vi "SwerveAntiDrift.vi"(1 "Max Driver Translation Joystick":dbl, 3 "Driver Rotation Joystick":dbl, 6 "PID Tuning Parameters":T1={"Kp"=0.1, "Ki"=0.1, "Kd"=0.1, "N-Diff"=10, "N-Int"=20, "Int Error Window"=0.5, "Max Ouput"=1.0, "Min Output"=-1.0, "Square Derivative"=FALSE, "N-Prop"=1} {"N-Prop" min=1; "Int Error Window" min=0.0; "N-Int" min=2; "N-Diff" min=2; "Kd" min=0.0; "Ki" min=0.0; "Kp" min=0.0}, 8 "Deceleration Hysteresis (ms)":u32, 10 "Strafe Deadband (ft/s)":dbl, 12 "External Disables":bool) -> (14 "Controller Summary":T2(graph), 17 "Joystick Rotation":dbl, 19 "Anti-Drift":bool)   [LabVIEW 2020]
doc: "This VI runs a PID controller to maintain the robot's heading while translating above a specified velocity. Dropping below the velocity threshold or manually commanding a rotation will switch off the anti-drift heading lock. Assumes that all of the joystick deadbands and scalings have already been applied."
uses:
  Globals/Sensor_Values.vi
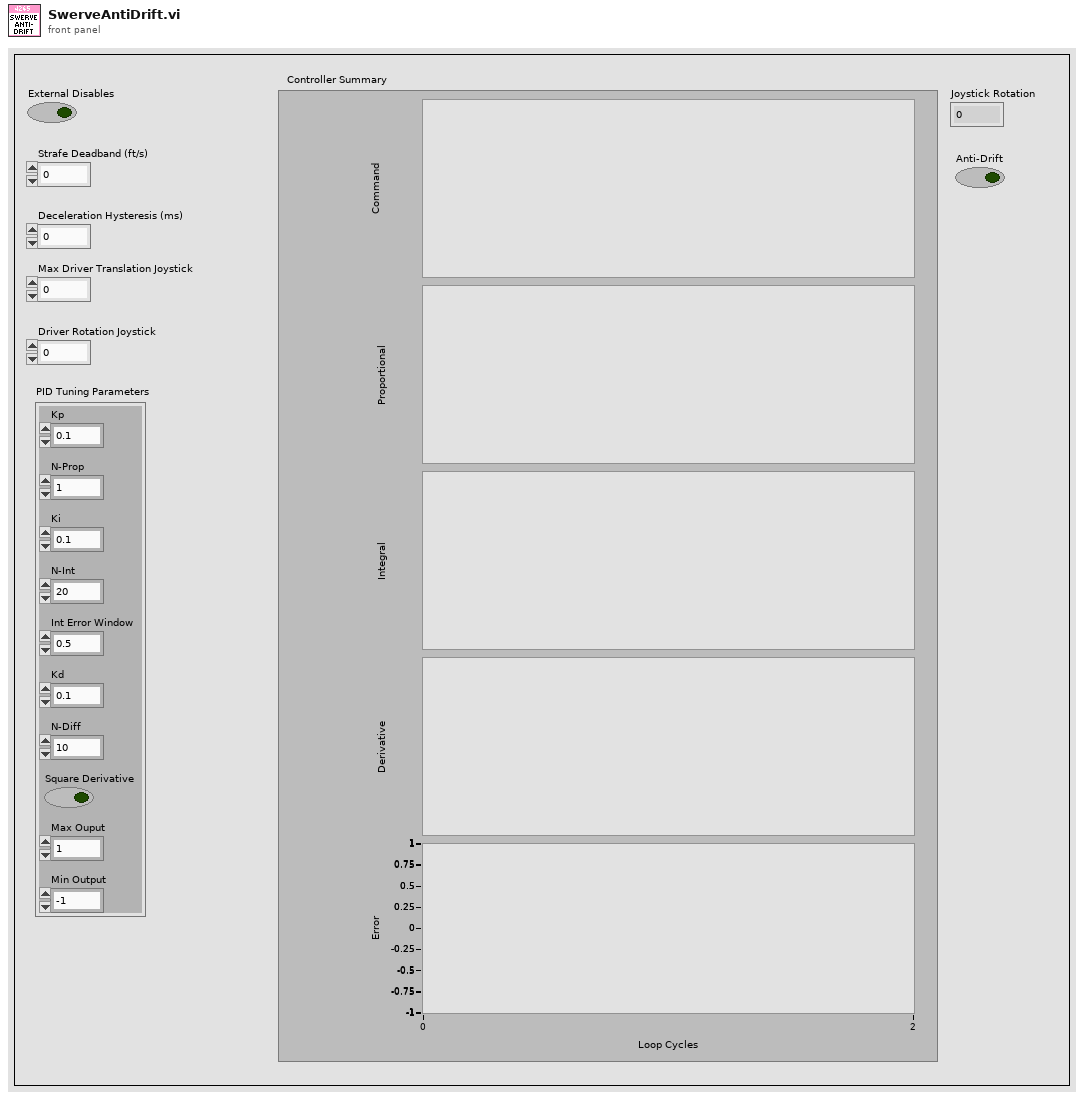
[diagram p1: front panel]
types:
  T1 = cluster{"Kp":dbl, "Ki":dbl, "Kd":dbl, "N-Diff":i32, "N-Int":i32, "Int Error Window":dbl, "Max Ouput":dbl, "Min Output":dbl, "Square Derivative":bool, "N-Prop":i32}
  T2 = cluster{"Command":dbl, "Proportional":dbl, "Integral":dbl, "Derivative":dbl, "Goal":dbl}
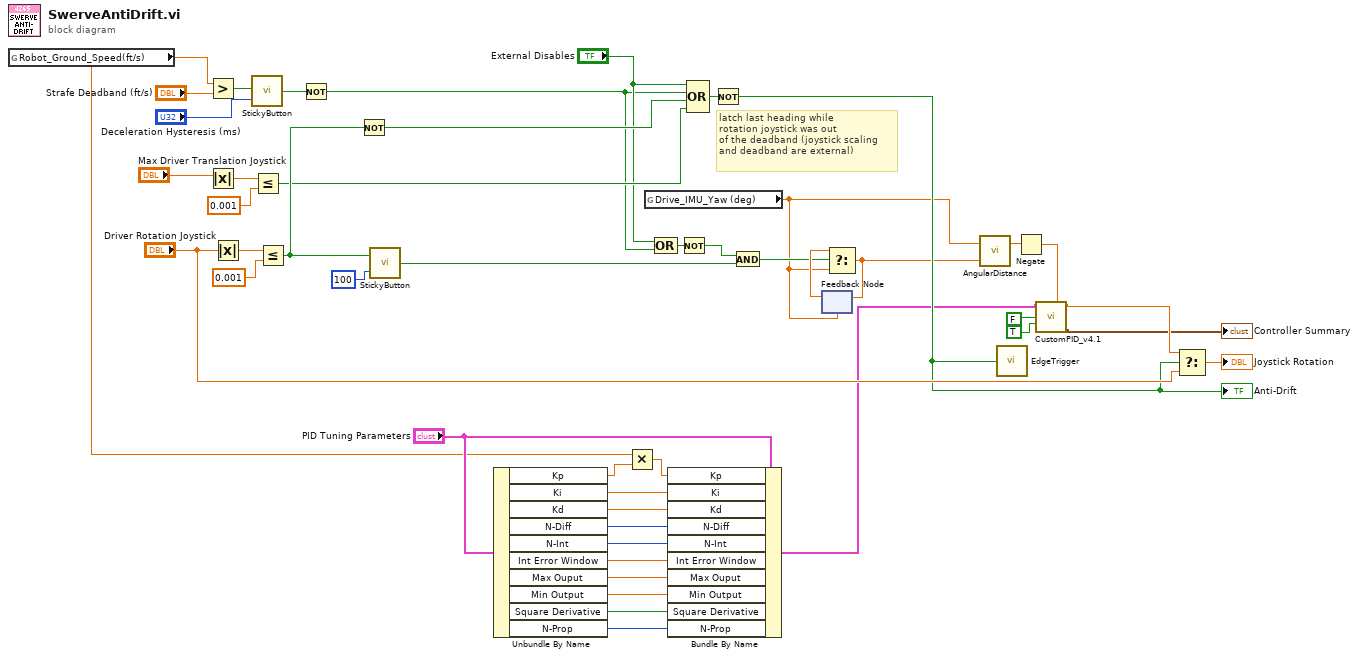
[diagram p0: block diagram]
diagram:
  # "latch last heading while\nrotation joystick was out \nof the deadband (joystick scaling \nand deadband are external)"
  n1 = global read "Sensor_Values.vi" "Robot_Ground_Speed(ft/s)"() -> (w10:dbl)
  n2 = Greater?(x=w10, y="Strafe Deadband (ft/s)") -> (0:w22:bool)
  n3 = Absolute Value(x="Max Driver Translation Joystick") -> (abs(x)=w20:dbl)
  n4 = Absolute Value(x="Driver Rotation Joystick") -> (abs(x)=w46:dbl)
  n5 = call "StickyButton.vi"("Time threshold (ms)"="Deceleration Hysteresis (ms)", "Button Input"=w22) -> ("Sticky Button"=w21:bool)
  n6 = Less Or Equal?(x=w20, y=0.001) -> (x <= y?=w17:bool)
  n7 = Less Or Equal?(x=w46, y=0.001) -> (x <= y?=w24:bool)
  n8 = Not(x=w21) -> (.not. x?=w15:bool)
  n9 = Not(x=w24) -> (.not. x?=w40:bool)
  n10 = call "StickyButton.vi"("Time threshold (ms)"=u32 100 ("y"), "Button Input"=w24) -> ("Sticky Button"=w36:bool)
  n11 = Unbundle By Name("PID Tuning Parameters") -> ("Kp"=w13:dbl, "Ki"=w11:dbl, "Kd"=w32:dbl, "N-Diff"=w31:i32, "N-Int"=w30:i32, "Int Error Window"=w29:dbl, "Max Ouput"=w28:dbl, "Min Output"=w27:dbl, "Square Derivative"=w26:bool, "N-Prop"=w25:i32)
  n12 = Multiply(x=w10, y=w13) -> (x*y=w12:dbl)
  n13 = global read "Sensor_Values.vi" "Drive_IMU_Yaw (deg)"() -> (w2:dbl)
  n14 = Compound Arithmetic op=OR("External Disables", w15) -> (w14:bool)
  n15 = Bundle By Name(cluster="PID Tuning Parameters", "Kp"=w12, "Ki"=w11, "Kd"=w32, "N-Diff"=w31, "N-Int"=w30, "Int Error Window"=w29, "Max Ouput"=w28, "Min Output"=w27, "Square Derivative"=w26, "N-Prop"=w25) -> (w9:T1)
  n16 = Not(x=w14) -> (.not. x?=w35:bool)
  n17 = Compound Arithmetic op=OR("External Disables", w15, w40, w17) -> (w39:bool)
  n18 = Not(x=w39) -> (.not. x?=w38:bool)
  "Anti-Drift" <- w38
  n19 = And(x=w35, y=w36) -> (x .and. y?=w34:bool)
  n20 = feedback #1(w2) -> (w41:dbl)
  n21 = Select(t=w41, s=w34, f=w2) -> (s? t:f=w1:dbl)
  n22 = feedback-in #1(w1) -> ()
  n23 = call "AngularDistance.vi"("Goal Angle (deg) [0,360]"=w1, "Current Angle (deg) [-Inf,+Inf]"=w2) -> ("Signed Angular Distance (deg) [-180,+180]"=w3:dbl)  [unwired: 1 out]
  n24 = call "EdgeTrigger.vi"("Input Signal"=w38) -> ()  [unwired: 3 out]
  n25 = Negate(x=w3) -> (-x=w4:dbl)
  n26 = call "CustomPID_v4.1.vi"("PID Tuning Parameters"=w9, "Custom Error Calculation"=w4, "Reset on Goal Change ?"=FALSE, "Use Custom Error Calculation ?"=TRUE) -> ("Command"=w8:dbl, "Controller Summary"=→"Controller Summary":T2)  [unwired: 8 in, 2 out]
  n27 = Select(t=w8, s=w38, f="Driver Rotation Joystick") -> (s? t:f=→"Joystick Rotation":dbl)
